vi "Set DC Voltage.vi"(8 "error in (no error)":errorcluster, 10 "Volt":dbl format="%.4f", 11 "Low Level PSU in":refnum<class "Low Level PSU.lvclass">) -> (0 "error out":errorcluster, 3 "Low Level PSU out":refnum<class "Low Level PSU.lvclass">)   [LabVIEW 2020, in "Low Level PSU With Tests.lvlib" / "Low Level PSU.lvclass"]
uses:
  Low Level PSU.lvclass
  Low Level PSU.lvclass/Low Level PSU.ctl
  Instrument Interface/Instrument Interface.lvclass
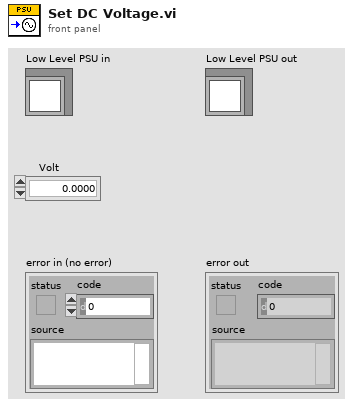
[diagram p1: front panel]
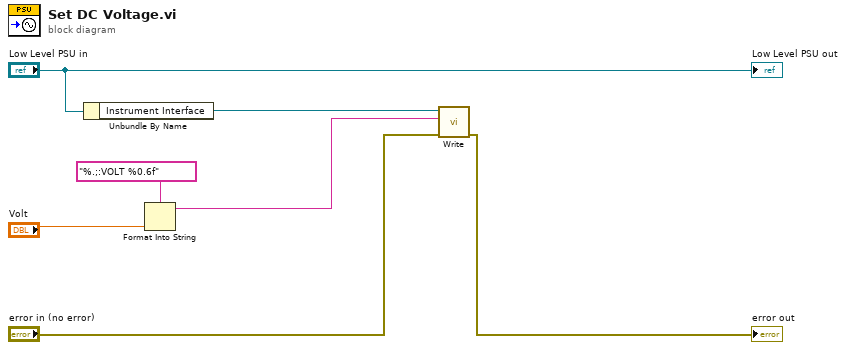
[diagram p0: block diagram]
diagram:
  n1 = Unbundle By Name("Low Level PSU in") -> ("Instrument Interface"=w4:refnum<class "Instrument Interface.lvclass">)
  n2 = Format Into String(format string="%.;:VOLT %0.6f", "Volt") -> (resulting string=w1:string)  [unwired: 2 in, 1 out]
  n3 = call-dynamic "Write.vi"("error in (no error)"="error in (no error)", "Data"=w1, "Instrument Interface in"=w4) -> ("error out"=→"error out":errorcluster)  [unwired: 7 in, 1 out]
  "Low Level PSU out" <- "Low Level PSU in"
